vi "Format to TmeStamp_Headers.vi"(8 "error in":errorcluster, 11 "String":string) -> (0 "error out":errorcluster, 3 "Time Stamp Out":timestamp format="%<%I:%M:%S%3u %p\n%m/%d/%Y>T")   [LabVIEW 2017, in "Data Operations.lvlib"]
uses:
  Data Operations.lvlib
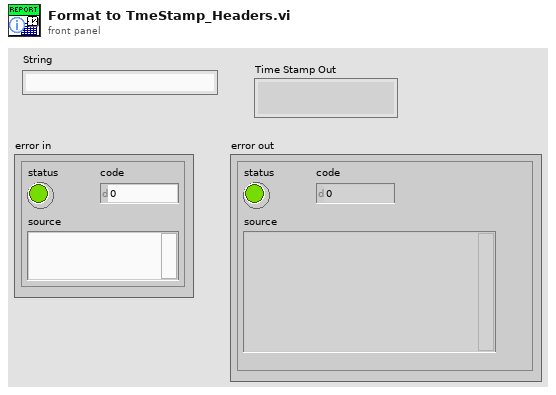
[diagram p1: front panel]
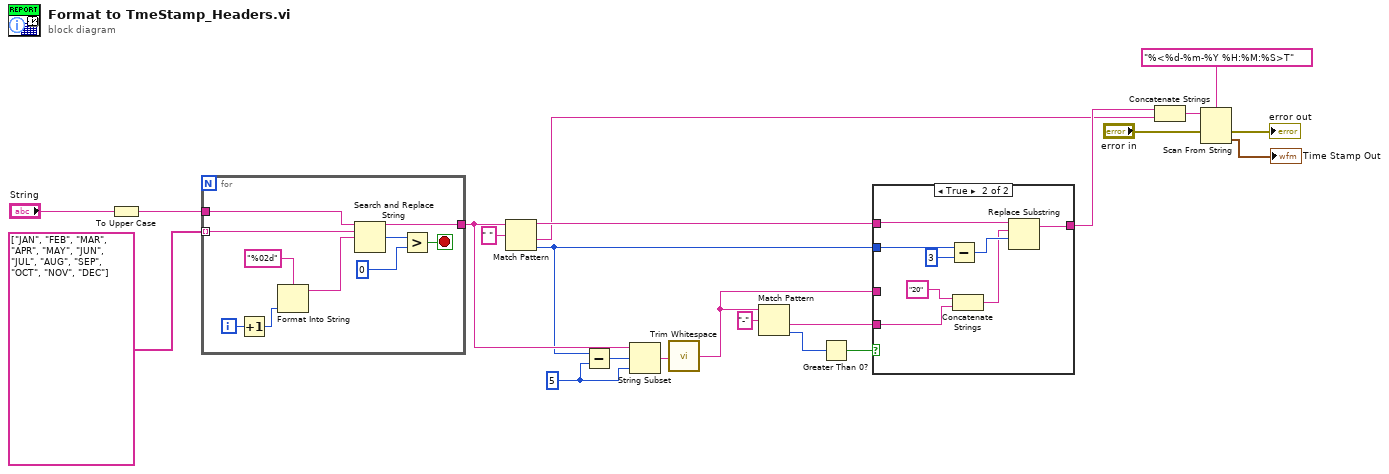
[diagram p0: block diagram]
diagram:
  w19 = 5 ("y")
  n1 = To Upper Case(1:"String") -> (0:w1:string)
  n2 = for {
    tunnel: w1 -> [w32]
    tunnel: string[] ["JAN", "FEB", "MAR", "APR", "MAY", "JUN", "JUL", "AUG", "SEP", "OCT", "NOV", "DEC"] -> [w31] mode=indexing
    tunnel: [w23] -> w20
    i -> [w30]
    stop <- w24 stop-if-true
    n3 = Increment(x=w30) -> (x+1=w29:i32)
    n4 = Format Into String(format string="%02d", w29) -> (resulting string=w27:string)  [unwired: 2 in, 1 out]
    n5 = Search and Replace String(input string=w32, search string=w31, replace string=w27) -> (result string=w23:string, number of replacements=w26:i32)  [unwired: 5 in, 2 out]
    n6 = Greater?(x=w26, y=0) -> (0:w24:bool)
  }
  n7 = Match Pattern(string=w20, regular expression=" ") -> (before substring=w11:string, after substring=w4:string, offset past match=w10:i32)  [unwired: 1 in, 1 out]
  n8 = Subtract(x=w10, y=w19) -> (x-y=w12:i32)
  n9 = String Subset(string=w20, offset (0)=w12, length (rest)=w19) -> (substring=w18:string)
  n10 = call <vilib>:"Trim Whitespace.vi"("string"=w18) -> ("trimmed string"=w13:string)  [unwired: 1 in]
  n11 = Match Pattern(string=w13, regular expression="-") -> (after substring=w15:string, offset past match=w16:i32)  [unwired: 1 in, 2 out]
  n12 = Greater Than 0?(x=w16) -> (x > 0?=w14:bool)
  n13 = case shown="True" w14 {
    tunnel: w15 -> [_ w40]
    tunnel: w13 -> [_ _]
    tunnel: w11 -> [w33 w39]
    tunnel: w10 -> [_ w38]
    tunnel: [w33 w34] -> w5
    frame False {
    }
    frame True {
      n14 = Subtract(x=w38, y=3) -> (x-y=w36:i32)
      n15 = Concatenate Strings("20" ("string"), w40) -> (w35:string)
      n16 = Replace Substring(3:w36, 4:w35, 5:w39) -> (1:w34:string)  [unwired: 1 in, 1 out]
    }
  }
  n17 = Concatenate Strings(w5, w4) -> (w3:string)
  n18 = Scan From String(format string="%<%d-%m-%Y %H:%M:%S>T", input string=w3, error in="error in") -> (error out=→"error out":errorcluster, output 1=→"Time Stamp Out":timestamp)  [unwired: 2 in, 2 out]
